vi "HIA_Query.vi"(0 "System no.":i32=1 min=1 max=4 step=1, 2 "Axes to query":string[](array[string]), 3 "Function":i32[](array[numeric]), 4 "All axes/functions?":bool, 5 "error in":errorcluster) -> (14 "DeviceID":i32[](array[numeric]), 15 "DeviceAxis":i32[](array[numeric]), 16 "Queried axes out":string[](array[string]), 17 "Function out":i32[](array[numeric]), 19 "error out":errorcluster)   [LabVIEW 2020]
doc: "This VI returns the current assignment of axes of Human Interface Devices (HID) to functions of controller axes and queries error. See controller user manual for details. Requires Build SPA query command substring.vi and Assign SPA values from string to axes.vi to be present. \n\nC-867: If All axes/functions? = FALSE, query is limited to up to one (.1*) / two (.2*) axes/functions per call.\n\nC-884: If All axes/functions? = FALSE, query is limited to up to 4 axes/functions per call.\n\nE-871, E-872, E-873: If All axes/functions? = FALSE, query is limited to one axis/function per call."
panel:
  # "This vi returns the current assignment of axes of Human Interface Devices (HID) to functions of controller \naxes and queries error. See controller User Manual for details.  Requires \"Build SPA query command \nsubstring.vi\" and \"Assign SPA values from string to axes.vi\" to be present."
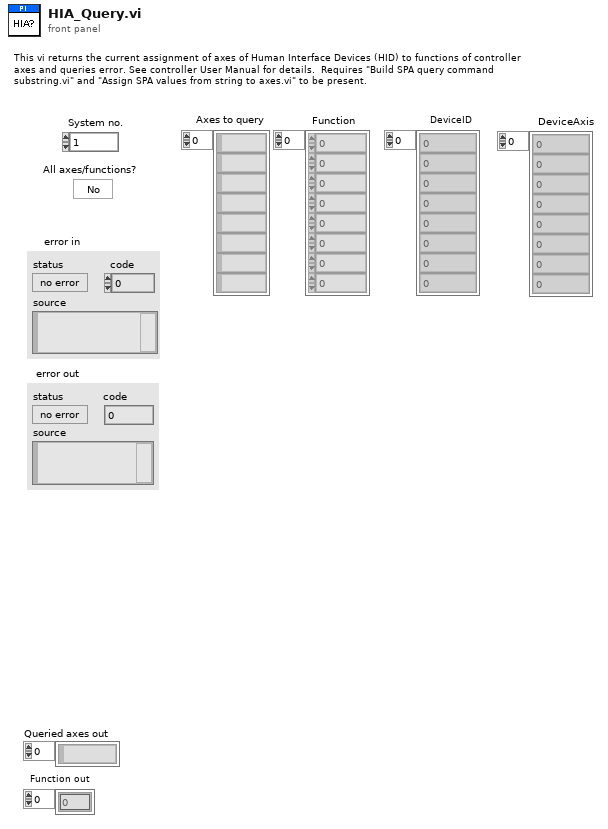
[diagram p1: front panel]
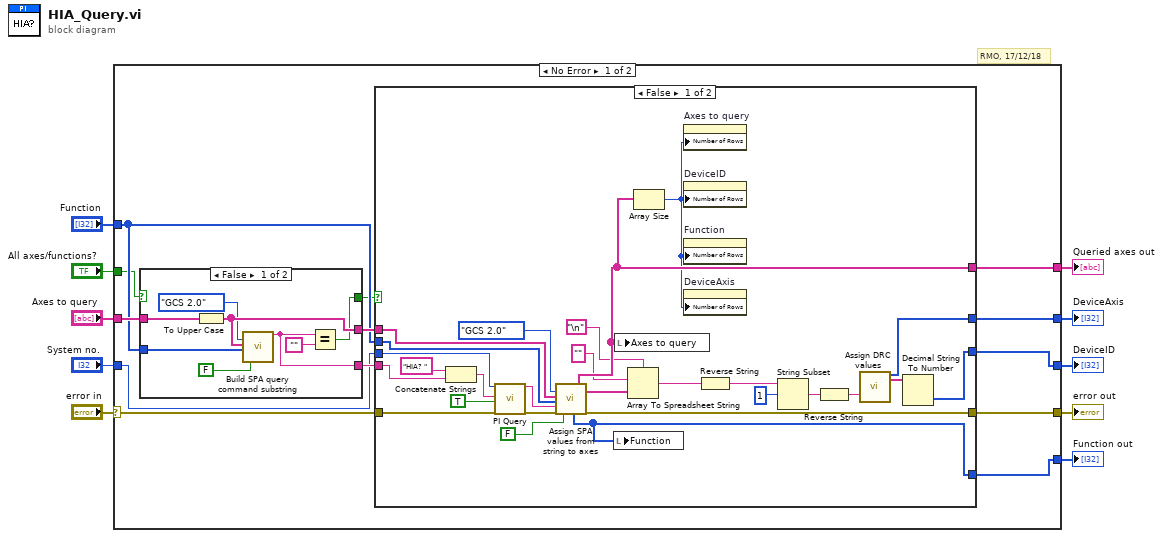
[diagram p0: block diagram]
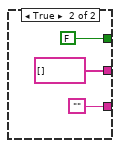
[diagram p2: hidden frame]
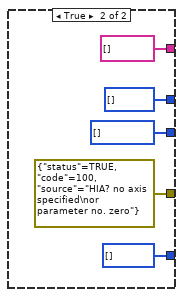
[diagram p3: hidden frame]
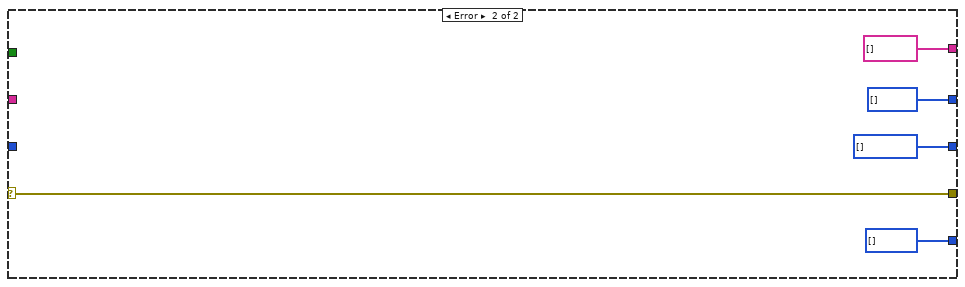
[diagram p4: hidden frame]
diagram:
  # "RMO, 17/12/18"
  n1 = case shown="No Error" "error in" {
    selector: "error in" -> [w11 w67]
    tunnel: "Axes to query" -> [w23 _]
    tunnel: "System no." -> [w14 _]
    tunnel: "Function" -> [w20 _]
    tunnel: [w19 w67] -> w7
    tunnel: [w17 i32[] [] ("Parameter values")] -> w6
    tunnel: "All axes/functions?" -> [w16 _]
    tunnel: [w15 i32[] [] ("Parameter strings")] -> w4
    tunnel: [w13 string[] [] ("Queried axes out")] -> w3
    tunnel: [w12 i32[] [] ("Parameter no. out")] -> w2
    frame No Error {
      n2 = case shown="False" w16 {
        tunnel: w23 -> [w31 _]
        tunnel: [w30 "" ("Command substring")] -> w22
        tunnel: [w29 string[] [] ("Designator to query")] -> w21
        tunnel: w20 -> [w28 _]
        tunnel: [w27 FALSE] -> w18
        frame False {
          n3 = To Upper Case(1:w31) -> (0:w29:string[])
          n4 = call "Build SPA query command substring.vi"("Syntax"=enum16{"GCS 1.0", "GCS 2.0"}."GCS 2.0", "Axes to query"=w29, "Parameter number"=w28, "Parameter no. format \n(Decimal: FALSE)"=FALSE ("Parameter no. format \n(Decimal: FALSE)")) -> ("Command substring"=w30:string)  [unwired: 3 in, 12 out]
          n5 = Equal?(x=w30, y="" ("x")) -> (x = y?=w27:bool)
        }
        frame True {
        }
      }
      n6 = case shown="False" w18 {
        tunnel: w11 -> [w55 _]
        tunnel: w22 -> [w58 _]
        tunnel: w21 -> [w57 _]
        tunnel: w14 -> [w40 _]
        tunnel: w20 -> [w56 _]
        tunnel: [w35 errorcluster {"status"=TRUE, "code"=100, "source"="HIA? no axis specified\nor parameter no. zero"} ("error out")] -> w19
        tunnel: [w39 i32[] [] ("Parameter values")] -> w17
        tunnel: [w38 i32[] [] ("Parameter strings")] -> w15
        tunnel: [w53 string[] [] ("Queried axes out")] -> w13
        tunnel: [w54 i32[] [] ("Parameter no. out")] -> w12
        frame False {
          n7 = Concatenate Strings("HIA? ", w58) -> (w59:string)
          n8 = call "PI Query.vi"("System no."=w40, "String to send"=w59, "Attach termination char.?"=TRUE ("Attach Linefeed?"), "error in"=w55) -> ("String read"=w37:string, "error out"=w36:errorcluster)  [unwired: 3 in, 11 out]
          n9 = call "Assign SPA values from string to axes.vi"("Syntax"=enum16{"GCS 1.0", "GCS 2.0"}."GCS 2.0", "Queried axes"=w57, "Parameter no."=w56, "Input string"=w37, "error in"=w36, "Parameter no. format \n(Decimal: FALSE)"=FALSE ("Parameter no. format \n(Decimal: FALSE)")) -> ("Parameter no. out"=w54:i32[], "Queried axes out"=w53:string[], "Parameter strings"=w42:string[], "error out"=w35:errorcluster)  [unwired: 2 in, 8 out]
          n10 = local write "Function"(w54) -> ()
          n11 = local write "Axes to query"(w53) -> ()
          n12 = Array To Spreadsheet String(delimiter (Tab)="\n", array=w42, 3:"" ("format string")) -> (spreadsheet string=w47:string)
          n13 = Array Size(array=w53) -> (size(s)=w52:i32)
          n14 = property on="Axes to query" class="Arr (strict)"("Number of Rows"=w52) -> ()  [unwired: 2 in, 2 out]
          n15 = property on="DeviceID" class="Arr (strict)"("Number of Rows"=w52) -> ()  [unwired: 2 in, 2 out]
          n16 = property on="Function" class="Arr (strict)"("Number of Rows"=w52) -> ()  [unwired: 2 in, 2 out]
          n17 = property on="DeviceAxis" class="Arr (strict)"("Number of Rows"=w52) -> ()  [unwired: 2 in, 2 out]
          n18 = Reverse String(1:w47) -> (0:w46:string)
          n19 = String Subset(string=w46, offset (0)=1) -> (substring=w44:string)  [unwired: 1 out]
          n20 = Reverse String(1:w44) -> (0:w43:string)
          n21 = call "Assign DRC values.vi"("Input String"=w43) -> ("Rec. option"=w38:i32[], "Source ID"=w41:string[])  [unwired: 2 in, 15 out]
          n22 = Decimal String To Number(string=w41) -> (number=w39:i32[])  [unwired: 3 out]
        }
        frame True {
        }
      }
    }
    frame Error {
    }
  }
  "error out" <- w7
  "DeviceID" <- w6
  "DeviceAxis" <- w4
  "Queried axes out" <- w3
  "Function out" <- w2
